vi "PID EGU to Percentage.vi"   [LabVIEW 2017, in "NI_PID_pid.lvlib"]
doc: "Converts an engineering-units input to a percent-of-range output based on the minimum and maximum range settings. Use the DBL instance of this VI to implement a single control loop. Use the DBL Array instance to implement parallel multi-loop control."
uses:
  <vilib>/addons/control/pid/NI_PID_pid.lvlib
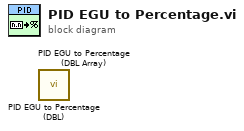
[diagram p0: block diagram]
diagram:
  n1 = call <vilib>:"PID EGU to Percentage (DBL).vi"() -> ()  [unwired: 3 in, 1 out]
  n2 = call <vilib>:"PID EGU to Percentage (DBL Array).vi"() -> ()  [unwired: 3 in, 1 out]
